vi "test Img.vi"() -> ()   [LabVIEW 2018, in "Image Process.lvclass"]
uses:
  Image Process.lvclass
panel:
  in  "Rectangle":T1
  out "Image":T2(plugin-control)
  out "error out":errorcluster
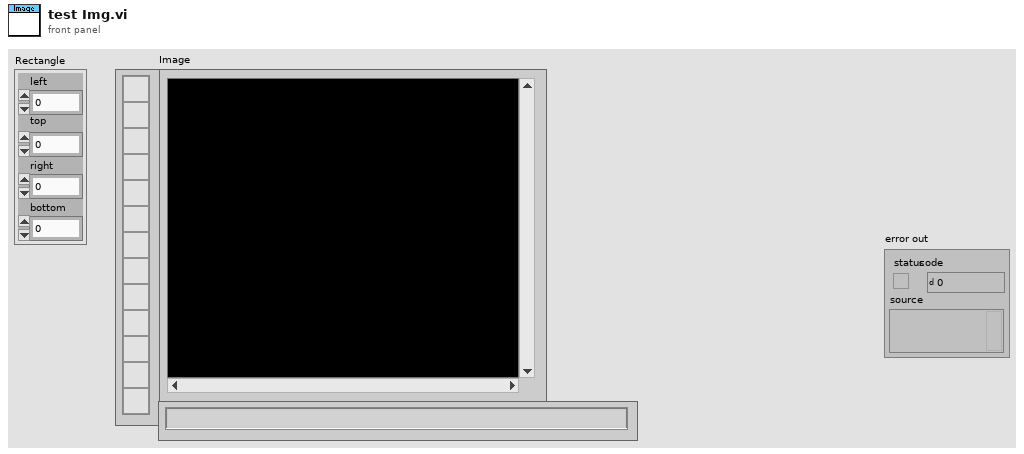
[diagram p1: front panel]
types:
  T1 = cluster{"left":i16, "top":i16, "right":i16, "bottom":i16}
  T2 = typedef "IMAQ Image.ctl" = refnum<image>
  T3 = typedef "Image Type" = u32
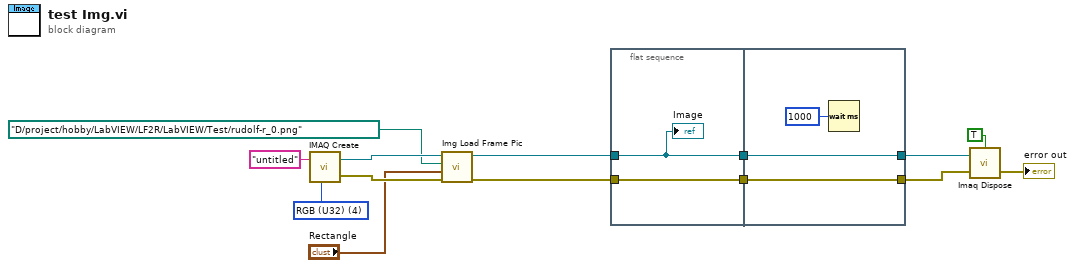
[diagram p0: block diagram]
diagram:
  w11 = T3 4 items=["Grayscale (U8)", "Grayscale (I16)", "Grayscale (SGL)", "Complex (CSG)", "RGB (U32)", "HSL (U32)", "RGB (U64)", "Grayscale (U16)"] ("Image Type")
  n1 = call "IMAQ Create"("Image Name"="untitled", "Image Type"=w11) -> ("New Image"=w4:T2, "error out"=w3:errorcluster)  [unwired: 3 in]
  n2 = call "Img Load Frame Pic.vi"("error in (no error)"=w3, "Rectangle"="Rectangle", "Image Path"=path "D:/project/hobby/LabVIEW/LF2R/LabVIEW/Test/rudolf-r_0.png" ("path to PNG file"), "Image In"=w4) -> ("error out"=w5:errorcluster, "Image Out"=w6:T2)  [unwired: 6 in]
  n3 = flat-sequence {
    tunnel: w6 -> [w15]
    tunnel: w5 -> [w16]
    tunnel: [w15] -> w14
    tunnel: [w16] -> w13
    tunnel: [w18] -> w8
    tunnel: [w19] -> w9
    tunnel: w14 -> [w19]
    tunnel: w13 -> [w18]
    frame #0 {
      "Image" <- w15
    }
    frame #1 {
      n4 = Wait (ms)(milliseconds to wait=u32 1000) -> ()  [unwired: 1 out]
    }
  }
  n5 = call "Imaq Dispose"("All Images? (No)"=TRUE, "Image"=w9, "error in (no error)"=w8) -> ("error out"=→"error out":errorcluster)  [unwired: 3 in]
